vi "Main.vi"() -> ()   [LabVIEW 2018, in "Impedance Tube.lvlib"]
uses:
  Impedance Tube.lvlib
  <vilib>/Analysis/6fits.llb/Remove Outliers (Index).vi
  <vilib>/Analysis/3filter.llb/Savitzky-Golay Filter (DBL).vi
  <vilib>/Utility/config.llb/Read Key (Boolean).vi
  <vilib>/Utility/config.llb/Read Key (Double).vi
  <vilib>/Utility/config.llb/Write Key (Boolean).vi
  <vilib>/Utility/config.llb/Write Key (Double).vi
  <vilib>/Utility/file.llb/Write Delimited Spreadsheet (DBL).vi
  <vilib>/Utility/config.llb/NI_LVConfig.lvlib
  <vilib>/Analysis/NI_AALPro.lvlib
  <vilib>/Analysis/NI_AALBase.lvlib
panel:
  out "Probe Calib Array":cdb[](array[numeric])
  out "max value 2":dbl
  out "max value":i32
  out "error":i32
  out "Filtered Alpha":dbl[](array[numeric])
  out "Normal Specific Impedence Ratio":cdb[](array[numeric])
  out "X Out":dbl[](array[numeric])
  out "Alpha Out":dbl[](array[numeric])
  in  "Mic Calibration":bool
  out "H":cdb[](array[numeric])
  in  "H1":cdb[](array[numeric])
  in  "H2":cdb[](array[numeric])
  in  "Store Params":bool
  in  "Tab Control":T1(tab)
  in  "Mic Device":dbl=4.0
  in  "Speaker Device":dbl
  out "Probe sensitivity ratio":dbl
  out "Upper Freq":dbl
  out "Probe Spacing":dbl
  out "Tube Diameter":dbl
  out "Frequency Spacing":dbl
  out "Speaker Hardware Error":bool
  out "Mic Hardware Error":bool
  out "Calibration Chart  2":dbl[](graph)
  out "Theta":dbl[](graph)
  out "Calibration Chart":cluster{i32, "df":dbl, dbl[]}(graph)
  out "H1 H2":cluster{i32, "df":dbl, "H2":dbl[]}[](graph)
  out "R 2":dbl[](graph)
  out "Alpha 2":cluster{"X Out":dbl[], "Y Out":dbl[]}(graph)
  out "Alpha 3":cluster{"X Out":dbl[], "Y Out":dbl[]}(graph)
  out "H1 H2 3":cluster{i32, dbl, dbl[]}(graph)
  out "R 3":dbl[](graph)
  out "H1 H2 2":cluster{i32, "df":dbl, "H2":dbl[]}[](graph)
  in  "Test Name":string
  in  "OK Button":bool
  out "Outlier Indexes":i32[](array[numeric])
  out "R":cdb[](array[numeric])
  out "Hbar":cdb[](array[numeric])
  in  "Measure":bool
  in  "H(c) 2":cdb[][](array[numeric])
  in  "H(c)":cdb[][](array[numeric])
  in  "output array":dbl[](array[numeric])
  out "Stsarted":bool
  in  "Mic 1 Device":dbl
  out "Mic A Device":dbl
  out "Speaker Volume":dbl
  out "s2 (mm)":dbl
  out "l (mm)":dbl
  out "s (mm)":dbl
  in  "Hardware Sync":bool
  in  "Sample Depth (mm)":dbl
  in  "Density of Air (kg/m3)":dbl
  in  "Speed of Sound m/s":dbl
  in  "Position":bool
  # "Control Panel"
  # "Mic A position"
  # "Position 1 \n(Low Frequency)"
  # "Position 2\n (High Frequency)"
  # "Note: \nSeal the empty mic hole"
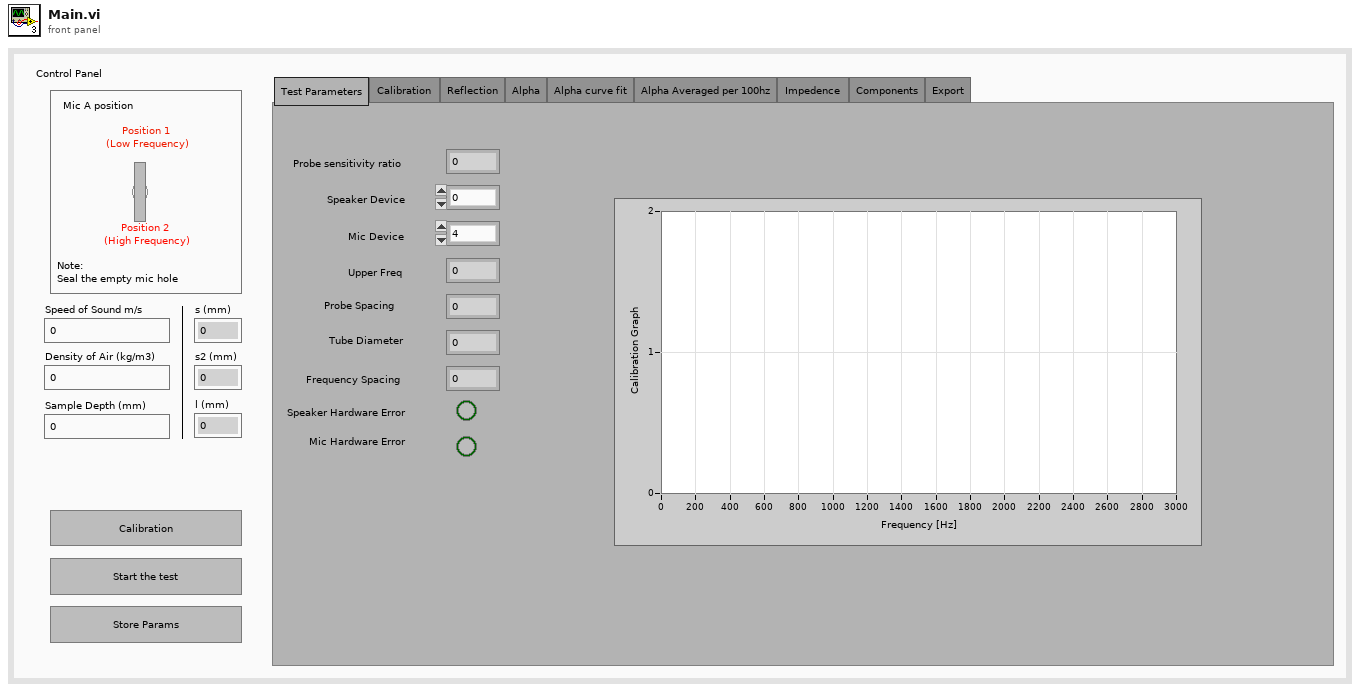
[diagram p1: front panel]
types:
  T1 = enum32{"Test Parameters", "Calibration ", "Reflection", "Alpha", "Alpha curve fit", "Alpha Averaged per 100hz", "Impedence ", "Components", "Export"}
  T2 = enum8{"Enabled", "Disabled", "Disabled and Grayed Out"}
  T3 = enum16{"open", "replace", "create", "open or create", "replace or create", "replace or create with confirmation"}
  T4 = typedef "NI_LVConfig.lvlib/Config Data RefNum.ctl" = refnum<k1>
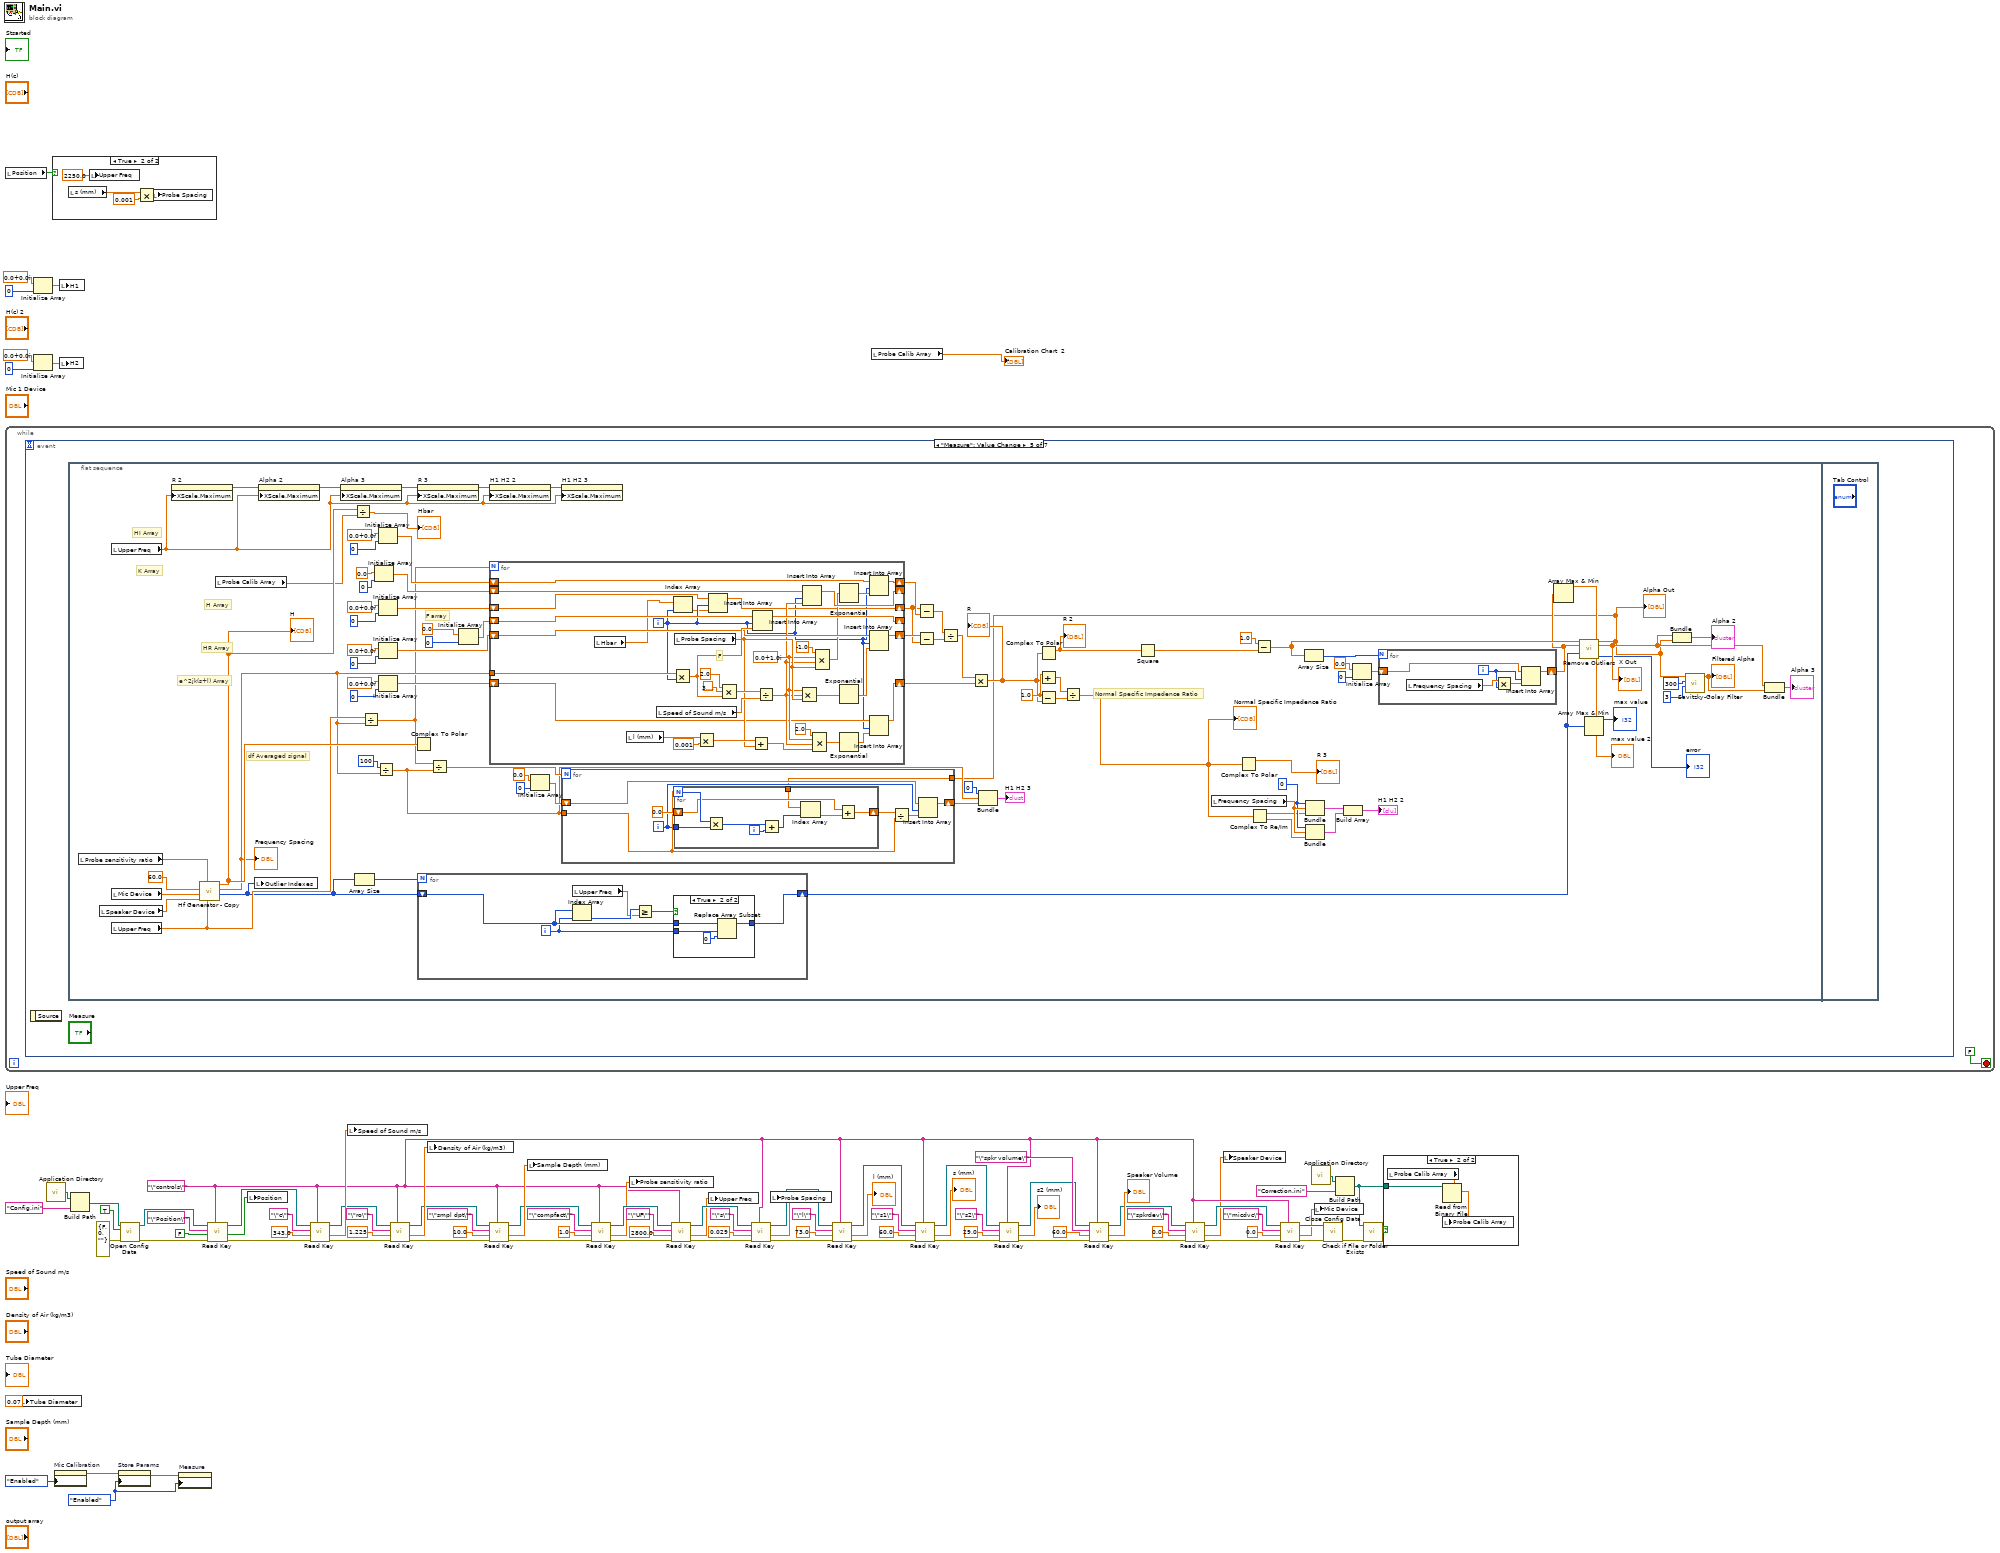
[diagram p0: block diagram]
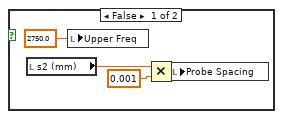
[diagram p2: hidden frame]
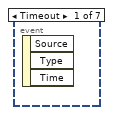
[diagram p4: hidden frame]
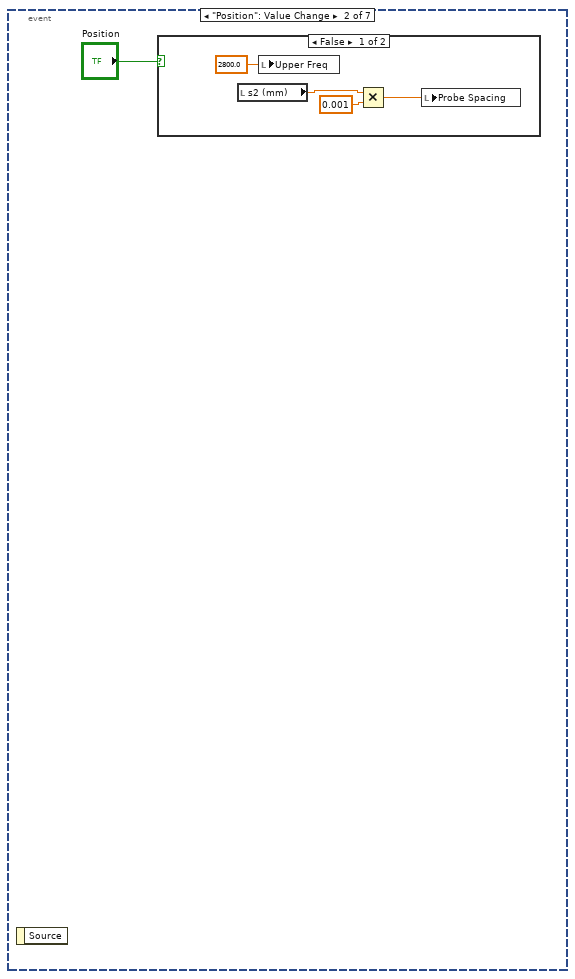
[diagram p5: hidden frame]
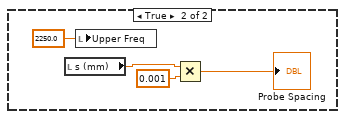
[diagram p6: hidden frame]
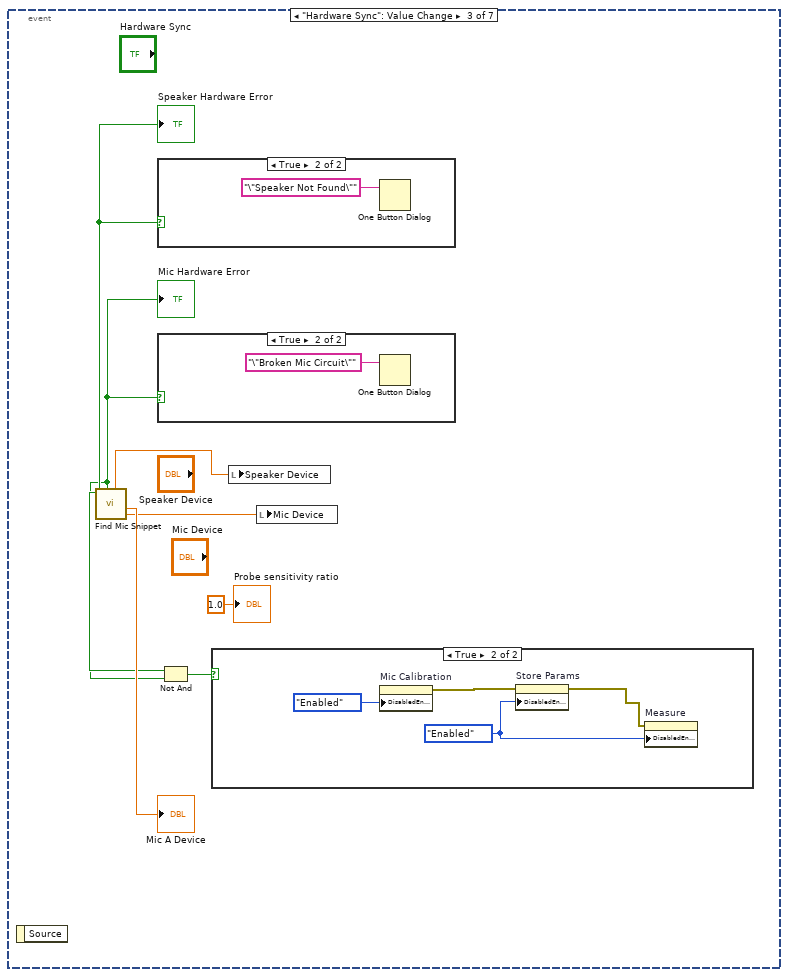
[diagram p7: hidden frame]
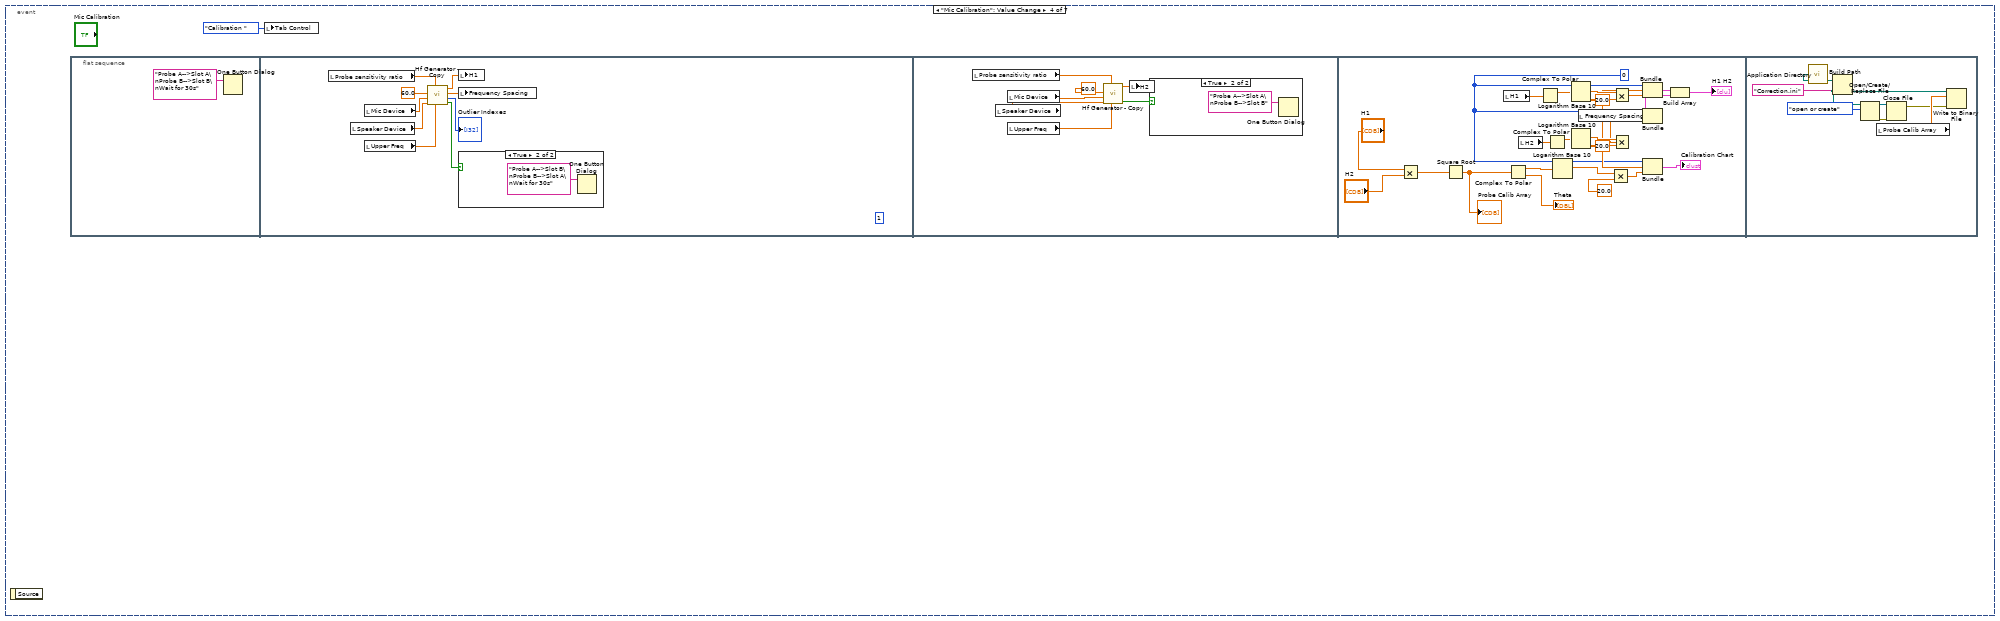
[diagram p11: hidden frame]
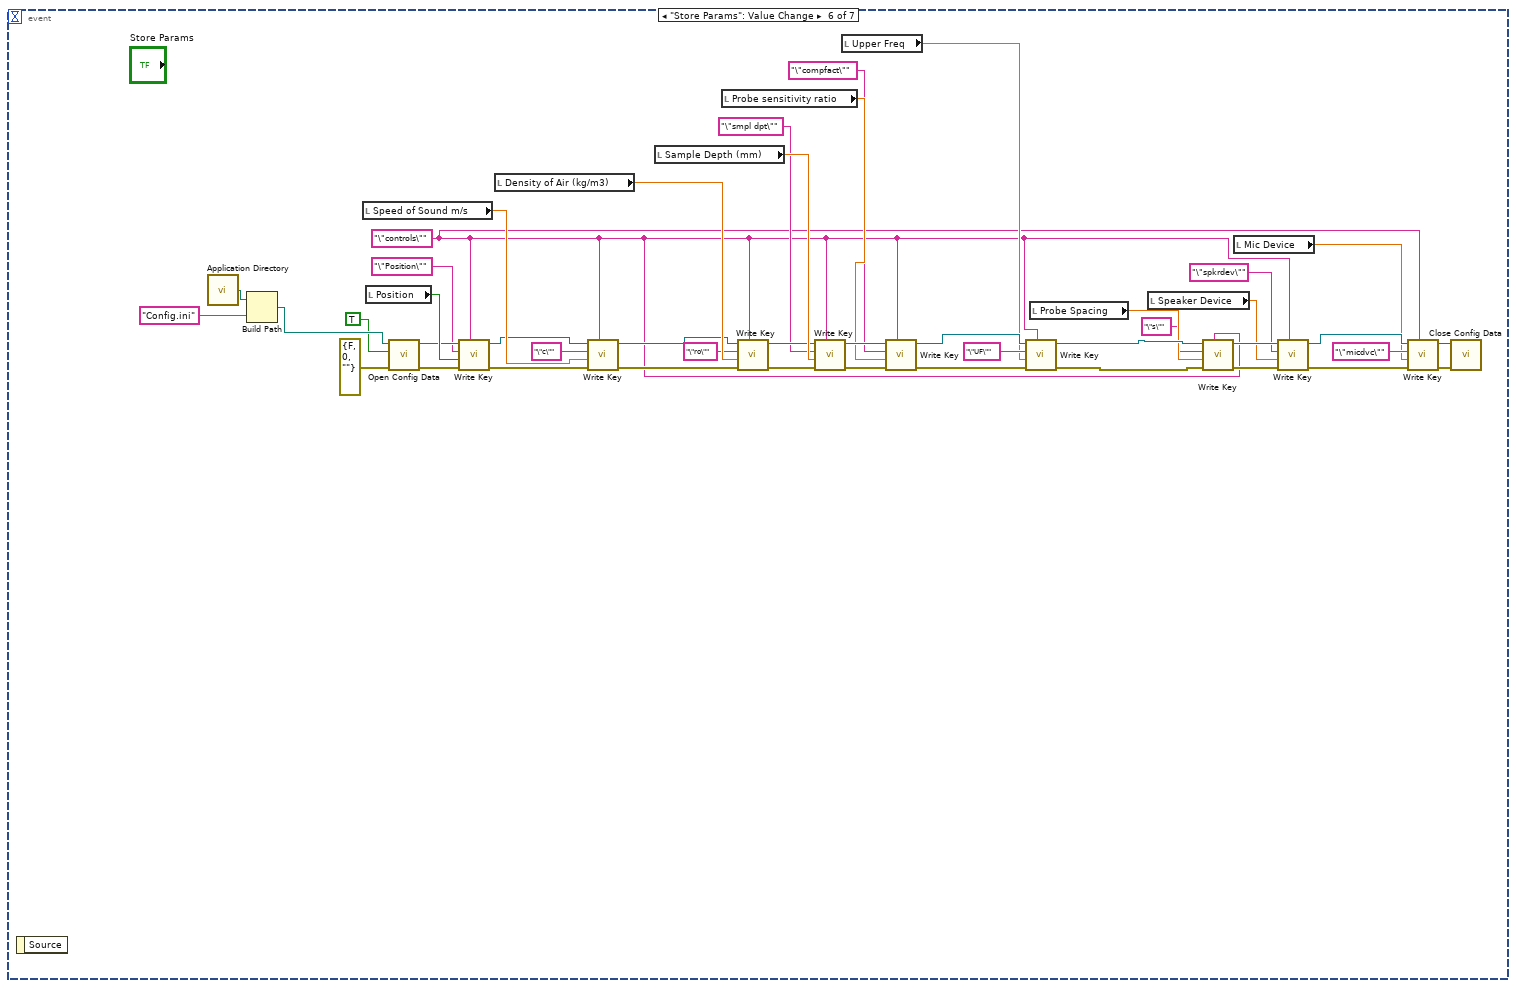
[diagram p15: hidden frame]
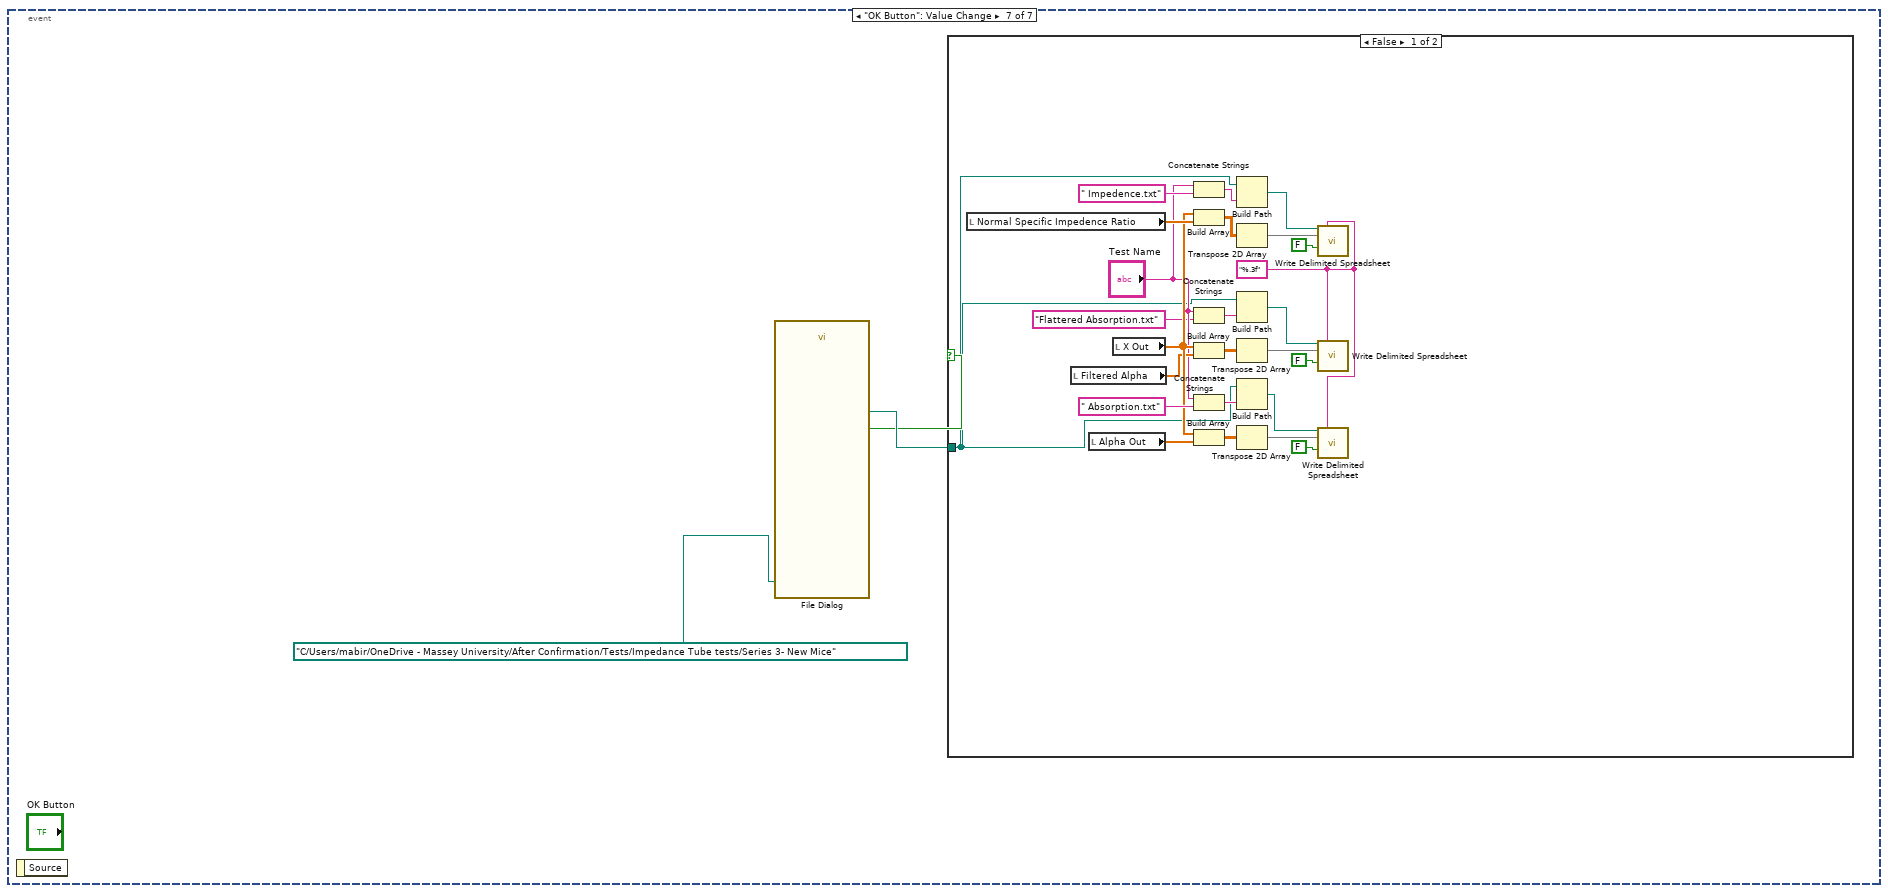
[diagram p16: hidden frame]
diagram:
  w1 = T2."Enabled" ("Disabled")
  w6 = "\"controls\"" ("section")
  n1 = local read "Position"() -> (w34:bool)
  n2 = while {
    stop <- FALSE stop-if-true
    n3 = event shown="[4] \"Measure\": Value Change" {
      selector: _ -> [_ _ _ _ _ _ _]
      dyn-events: _ -> [_ _ _ _ _ _ _]
      timeout: _ -> [_ _ _ _ _ _ _]
      event Timeout {
        n4 = event-data() -> ()  [unwired: 1 in, 3 out]
      }
      event "Position": Value Change {
        n5 = event-data() -> ()  [unwired: 1 in, 1 out]
        n6 = case shown="False" "Position" {
          frame False {
            n7 = local read "s2 (mm)"() -> (w96:dbl)
            n8 = local write "Upper Freq"(2800.0 ("Upper Freq")) -> ()
            n9 = Multiply(x=w96, y=0.001) -> (x*y=w95:dbl)
            n10 = local write "Probe Spacing"(w95) -> ()
          }
          frame True {
            n11 = local read "s (mm)"() -> (w100:dbl)
            n12 = local write "Upper Freq"(2250.0 ("Upper Freq")) -> ()
            n13 = Multiply(x=w100, y=0.001) -> (x*y=→"Probe Spacing":dbl)
          }
        }
      }
      event "Hardware Sync": Value Change {
        n14 = event-data() -> ()  [unwired: 1 in, 1 out]
        n15 = call "Find Mic Snippet.vi"() -> ("Mic B Device"=w103:dbl, "Mic A Device"=→"Mic A Device":dbl, "Speaker Device"=w102:dbl, "Faulty Mic"=w106:bool, "Speaker Not Found"=w107:bool)  [unwired: 3 in, 3 out]
        "Mic Hardware Error" <- w106
        "Speaker Hardware Error" <- w107
        n16 = case shown="True" w107 {
          frame False {
          }
          frame True {
            n17 = One Button Dialog(message="\"Speaker Not Found\"") -> ()  [unwired: 1 in, 1 out]
          }
        }
        n18 = case shown="True" w106 {
          frame False {
          }
          frame True {
            n19 = One Button Dialog(message="\"Broken Mic Circuit\"") -> ()  [unwired: 1 in, 1 out]
          }
        }
        n20 = Not And(1:w106, 2:w107) -> (0:w105:bool)
        n21 = case shown="True" w105 {
          frame False {
          }
          frame True {
            w109 = T2."Enabled" ("Disabled")
            n22 = property on="Mic Calibration" class="Bool"("DisabledEnum"=T2."Enabled" ("Disabled")) -> (error out=w111:errorcluster)  [unwired: 2 in, 1 out]
            n23 = property on="Store Params" class="Bool"(error in=w111, "DisabledEnum"=w109) -> (error out=w110:errorcluster)  [unwired: 1 in, 1 out]
            n24 = property on="Measure" class="Bool"(error in=w110, "DisabledEnum"=w109) -> ()  [unwired: 1 in, 2 out]
          }
        }
        n25 = local write "Speaker Device"(w102) -> ()
        n26 = local write "Mic Device"(w103) -> ()
        "Probe sensitivity ratio" <- 1.0 ("Probe sensitivity ratio")
      }
      event "Mic Calibration": Value Change {
        n27 = event-data() -> ()  [unwired: 1 in, 1 out]
        n28 = flat-sequence {
          frame #0 {
            n29 = One Button Dialog(message="Probe A-->Slot A\nProbe B-->Slot B\nWait for 30s") -> ()  [unwired: 1 in, 1 out]
          }
          frame #1 {
            (unwired) 1 ("Averages")
            n30 = local read "Probe sensitivity ratio"() -> (w122:dbl)
            n31 = local read "Speaker Device"() -> (w124:dbl)
            n32 = local read "Mic Device"() -> (w119:dbl)
            n33 = local read "Upper Freq"() -> (w121:dbl)
            n34 = call "Hf Generator - Copy.vi"("Upper Frequency"=w121, "Mic B Comp Fact"=w122, "Speaker Device"=w124, "Mic B"=w119, "Duration"=60.0) -> ("Done"=w120:bool, "Outlier Indexes"=→"Outlier Indexes":i32[], "df"=w117:dbl, "H(f)"=w123:cdb[])  [unwired: 1 in]
            n35 = local write "H1"(w123) -> ()
            n36 = local write "Frequency Spacing"(w117) -> ()
            n37 = case shown="True" w120 {
              frame False {
              }
              frame True {
                n38 = One Button Dialog(message="Probe A-->Slot B\nProbe B-->Slot A\nWait for 30s") -> ()  [unwired: 1 in, 1 out]
              }
            }
          }
          frame #2 {
            n39 = local read "Probe sensitivity ratio"() -> (w129:dbl)
            n40 = local read "Speaker Device"() -> (w131:dbl)
            n41 = local read "Mic Device"() -> (w133:dbl)
            n42 = local read "Upper Freq"() -> (w127:dbl)
            n43 = call "Hf Generator - Copy.vi"("Upper Frequency"=w127, "Mic B Comp Fact"=w129, "Speaker Device"=w131, "Mic B"=w133, "Duration"=60.0) -> ("Done"=w130:bool, "H(f)"=w128:cdb[])  [unwired: 1 in, 2 out]
            n44 = local write "H2"(w128) -> ()
            n45 = case shown="True" w130 {
              frame False {
              }
              frame True {
                n46 = One Button Dialog(message="Probe A-->Slot A\nProbe B-->Slot B") -> ()  [unwired: 1 in, 1 out]
              }
            }
          }
          frame #3 {
            w148 = 0
            n47 = Multiply(x="H1", y="H2") -> (x*y=w157:cdb[])
            n48 = Square Root(x=w157) -> (sqrt(x)=w135:cdb[])
            "Probe Calib Array" <- w135
            n49 = local read "H1"() -> (w153:cdb[])
            n50 = Complex To Polar(r * e^(i*theta)=w135) -> (r=w145:dbl[], theta=→"Theta":dbl[])
            n51 = local read "H2"() -> (w150:cdb[])
            n52 = Complex To Polar(r * e^(i*theta)=w153) -> (r=w140:dbl[])  [unwired: 1 out]
            n53 = Complex To Polar(r * e^(i*theta)=w150) -> (r=w139:dbl[])  [unwired: 1 out]
            n54 = Logarithm Base 10(1:w145) -> (0:w144:dbl[])
            n55 = Logarithm Base 10(1:w140) -> (0:w155:dbl[])
            n56 = Logarithm Base 10(1:w139) -> (0:w152:dbl[])
            n57 = local read "Frequency Spacing"() -> (w149:dbl)
            n58 = Multiply(x=w144, y=20.0) -> (x*y=w138:dbl[])
            n59 = Multiply(x=w155, y=20.0) -> (x*y=w154:dbl[])
            n60 = Multiply(x=w152, y=20.0) -> (x*y=w151:dbl[])
            n61 = Bundle(w148, "Frequency Spacing"=w149, w154) -> (w147:cluster{i32, "Frequency Spacing":dbl, dbl[]})  [unwired: 1 in]
            n62 = Bundle(w148, "Frequency Spacing"=w149, w151) -> (w146:cluster{i32, "Frequency Spacing":dbl, dbl[]})  [unwired: 1 in]
            n63 = Bundle(w148, "Frequency Spacing"=w149, w138) -> (→"Calibration Chart":cluster{i32, "Frequency Spacing":dbl, dbl[]})  [unwired: 1 in]
            n64 = Build Array(w147, w146) -> (→"H1 H2":cluster{i32, "Frequency Spacing":dbl, dbl[]}[])
          }
          frame #4 {
            n65 = call <vilib>:"Application Directory.vi"() -> ("Application Directory"=w167:path)
            n66 = Build Path(base path=w167, name or relative path="Correction.ini") -> (appended path=w163:path)
            n67 = Open/Create/Replace File(file path (use dialog)=w163, operation (0:open)=T3."open or create") -> (refnum out=w164:refnum<file>, error out=w162:errorcluster)  [unwired: 4 in, 1 out]
            n68 = local read "Probe Calib Array"() -> (w165:cdb[])
            n69 = Close File(refnum=w164, error in=w162) -> (error out=w161:errorcluster)  [unwired: 1 out]
            n70 = Write to Binary File(file (use dialog)=w163, data=w165, error in=w161) -> ()  [unwired: 3 in, 3 out]
          }
        }
        n71 = local write "Tab Control"(T1."Calibration " ("Tab Control")) -> ()
      }
      event "Measure": Value Change {
        n72 = event-data() -> ()  [unwired: 1 in, 1 out]
        n73 = flat-sequence {
          frame #0 {
            w186 = 0
            w192 = 1.0 ("x")
            # "Normal Specific Impedence Ratio"
            # "df Averaged signal"
            # "H Array"
            # "e^2jk(s+l) Array"
            # "HR Array"
            # "HI Array"
            # "K Array"
            # "F array"
            n74 = local read "Probe sensitivity ratio"() -> (w249:dbl)
            n75 = local read "Speaker Device"() -> (w250:dbl)
            n76 = local read "Upper Freq"() -> (w175:dbl)
            n77 = local read "Mic Device"() -> (w251:dbl)
            n78 = local read "Upper Freq"() -> (w244:dbl)
            n79 = property on="R 2" class="WFGraph (strict)"("XScale.Maximum"=w175) -> (error out=w180:errorcluster)  [unwired: 2 in, 1 out]
            n80 = call "Hf Generator - Copy.vi"("Upper Frequency"=w244, "Mic B Comp Fact"=w249, "Speaker Device"=w250, "Mic B"=w251, "Duration"=60.0) -> ("Outlier Indexes"=w199:i32[], "df"=w216:dbl, "H(f)"=w248:cdb[])  [unwired: 1 in, 1 out]
            "H" <- w248
            "Frequency Spacing" <- w216
            n81 = local read "Probe Calib Array"() -> (w247:cdb[])
            n82 = local write "Outlier Indexes"(w199) -> ()
            n83 = property on="Alpha 2" class="XYGraph (strict)"(error in=w180, "XScale.Maximum"=w175) -> (error out=w179:errorcluster)  [unwired: 1 in, 1 out]
            n84 = property on="Alpha 3" class="XYGraph (strict)"(error in=w179, "XScale.Maximum"=w175) -> (error out=w178:errorcluster)  [unwired: 1 in, 1 out]
            n85 = Divide(x=w248, y=w247) -> (x/y=→"Hbar":cdb[])
            n86 = Array Size(array=w199) -> (size(s)=w200:i32)
            n87 = Divide(x=w244, y=w216) -> (x/y=w215:dbl)
            n88 = Initialize Array(0.0 ("element"), 0 ("dimension size")) -> (w240:dbl[])
            n89 = Divide(x=100, y=w216) -> (x/y=w212:dbl)
            n90 = Initialize Array(cdb 0.0+0.0i ("complex element"), 0 ("dimension size")) -> (w235:cdb[])
            n91 = Initialize Array(cdb 0.0+0.0i ("complex element 4"), 0 ("dimension size")) -> (w222:cdb[])
            n92 = Initialize Array(cdb 0.0+0.0i ("complex element 2"), 0 ("dimension size")) -> (w234:cdb[])
            n93 = Initialize Array(cdb 0.0+0.0i ("complex element 3"), 0 ("dimension size")) -> (w231:cdb[])
            n94 = Complex To Polar(r * e^(i*theta)=w248) -> ()  [unwired: 2 out]
            n95 = property on="R 3" class="WFGraph (strict)"(error in=w178, "XScale.Maximum"=w175) -> (error out=w177:errorcluster)  [unwired: 1 in, 1 out]
            n96 = for {
              N: w200 -> [_]
              shift-right: [w253] -> w173
              shift-left: w199 -> [w255]
              i -> [w254]
              n97 = Index Array(array=w255, index=w254) -> (element=w258:i32)
              n98 = local read "Upper Freq"() -> (w257:dbl)
              n99 = Greater Or Equal?(x=w258, y=w257) -> (x >= y?=w256:bool)
              n100 = case shown="True" w256 {
                tunnel: w255 -> [w259 w263]
                tunnel: w254 -> [_ w262]
                tunnel: [w259 w260] -> w253
                frame False {
                }
                frame True {
                  n101 = Replace Array Subset(array=w263, new element=0 ("new element/subarray"), index=w262) -> (w260:i32[])
                }
              }
            }
            n102 = Divide(x=w215, y=w212) -> (x/y=w214:dbl)
            n103 = Initialize Array(0.0 ("element"), 0 ("dimension size")) -> (w243:dbl[])
            n104 = property on="H1 H2 2" class="WFGraph (strict)"(error in=w177, "XScale.Maximum"=w175) -> (error out=w176:errorcluster)  [unwired: 1 in, 1 out]
            n105 = for {
              N: w215 -> [_]
              shift-right: [w320] -> _
              shift-left: w243 -> [w321]
              tunnel: w216 -> [w319]
              shift-right: [w312] -> _
              shift-left: w240 -> [w313]
              shift-right: [w310] -> w230
              shift-left: w235 -> [w311]
              shift-right: [w308] -> w229
              shift-left: w234 -> [w309]
              shift-right: [w291] -> w225
              shift-left: w231 -> [w292]
              shift-right: [w289] -> w221
              shift-left: w222 -> [w290]
              i -> [w288]
              w297 = cdb 0.0+1.0i ("i")
              # "F"
              n106 = local read "Hbar"() -> (w286:cdb[])
              n107 = local read "l (mm)"() -> (w302:dbl)
              n108 = local read "Speed of Sound m/s"() -> (w314:dbl)
              n109 = Multiply(x=w319, y=w288) -> (x*y=w316:dbl)
              n110 = Index Array(array=w286, index=w288) -> (element=w287:cdb)
              n111 = local read "Probe Spacing"() -> (w299:dbl)
              n112 = Multiply(x=w302, y=0.001) -> (x*y=w300:dbl)
              n113 = Insert Into Array(array=w290, index=w288, new element=w287) -> (w289:cdb[])
              n114 = Compound Arithmetic op=MULTIPLY(2.0 ("value"), 3.141592653589793, w316) -> (w315:dbl)
              n115 = Add(x=w300, y=w299) -> (x+y=w295:dbl)
              n116 = Insert Into Array(array=w321, index=w288, new element=w316) -> (w320:dbl[])
              n117 = Divide(x=w315, y=w314) -> (x/y=w296:dbl)
              n118 = Insert Into Array(array=w313, index=w288, new element=w296) -> (w312:dbl[])
              n119 = Compound Arithmetic op=MULTIPLY(w297, w296, w299) -> (w304:cdb)
              n120 = Compound Arithmetic op=MULTIPLY(2.0 ("value"), w297, w296, w295) -> (w294:cdb)
              n121 = Compound Arithmetic op=MULTIPLY(-1.0 ("value"), w297, w296, w299) -> (w306:cdb)
              n122 = Exponential(1:w306) -> (0:w305:cdb)
              n123 = Exponential(1:w304) -> (0:w303:cdb)
              n124 = Exponential(1:w294) -> (0:w293:cdb)
              n125 = Insert Into Array(array=w311, index=w288, new element=w305) -> (w310:cdb[])
              n126 = Insert Into Array(array=w309, index=w288, new element=w303) -> (w308:cdb[])
              n127 = Insert Into Array(array=w292, index=w288, new element=w293) -> (w291:cdb[])
            }
            n128 = Initialize Array(0.0 ("element"), 0 ("dimension size")) -> (w218:dbl[])
            n129 = property on="H1 H2 3" class="WFGraph (strict)"(error in=w176, "XScale.Maximum"=w175) -> ()  [unwired: 1 in, 2 out]
            n130 = Subtract(x=w221, y=w230) -> (x-y=w228:cdb[])
            n131 = Subtract(x=w229, y=w221) -> (x-y=w227:cdb[])
            n132 = Divide(x=w228, y=w227) -> (x/y=w226:cdb[])
            n133 = Multiply(x=w226, y=w225) -> (x*y=w191:cdb[])
            "R" <- w191
            n134 = Add(x=w192, y=w191) -> (x+y=w193:cdb[])
            n135 = Subtract(x=w192, y=w191) -> (x-y=w190:cdb[])
            n136 = Complex To Polar(r * e^(i*theta)=w191) -> (r=w208:dbl[])  [unwired: 1 out]
            "R 2" <- w208
            n137 = Divide(x=w193, y=w190) -> (x/y=w189:cdb[])
            "Normal Specific Impedence Ratio" <- w189
            n138 = Square(x=w208) -> (x^2=w207:dbl[])
            n139 = local read "Frequency Spacing"() -> (w187:dbl)
            n140 = Complex To Polar(r * e^(i*theta)=w189) -> (r=→"R 3":dbl[])  [unwired: 1 out]
            n141 = Complex To Re/Im(x + iy=w189) -> (x=w184:dbl[], y=w185:dbl[])
            n142 = Subtract(x=1.0, y=w207) -> (x-y=w202:dbl[])
            n143 = Array Size(array=w202) -> (size(s)=w206:i32)
            n144 = Bundle(w186, "Frequency Spacing"=w187, w184) -> (w182:cluster{i32, "Frequency Spacing":dbl, dbl[]})  [unwired: 1 in]
            n145 = Bundle(w186, "Frequency Spacing"=w187, w185) -> (w183:cluster{i32, "Frequency Spacing":dbl, dbl[]})  [unwired: 1 in]
            n146 = Build Array(w182, w183) -> (→"H1 H2 2":cluster{i32, "Frequency Spacing":dbl, dbl[]}[])
            n147 = Initialize Array(0.0 ("element"), 0 ("dimension size")) -> (w203:dbl[])
            n148 = for {
              N: w206 -> [_]
              shift-right: [w266] -> w171
              shift-left: w203 -> [w267]
              i -> [w265]
              n149 = local read "Frequency Spacing"() -> (w268:dbl)
              n150 = Multiply(x=w268, y=w265) -> (x*y=w264:dbl)
              n151 = Insert Into Array(array=w267, index=w265, new element=w264) -> (w266:dbl[])
            }
            n152 = Array Max & Min(array=w171) -> (max value=→"max value 2":dbl)  [unwired: 3 out]
            n153 = call-poly <vilib>:"Remove Outliers.vi"("Y"=w202, "X"=w171, "Index"=w173) -> ("Y Out"=w168:dbl[], "X Out"=w198:dbl[], "error"=→"error":i32)  [unwired: 9 in, 1 out]
            "Alpha Out" <- w168
            "X Out" <- w198
            n154 = for {
              N: w214 -> [_]
              shift-right: [w272] -> w213
              shift-left: w218 -> [w273]
              tunnel: w212 -> [w274]
              tunnel: w168 -> [w269]
              i -> [w271]
              n155 = for {
                N: w274 -> [w284]
                tunnel: w271 -> [w285]
                shift-right: [w279] -> w275
                shift-left: 0.0 ("element") -> [w280]
                tunnel: w269 -> [w277]
                i -> [w282]
                n156 = Multiply(x=w284, y=w285) -> (x*y=w283:i32)
                n157 = Add(x=w283, y=w282) -> (x+y=w281:i32)
                n158 = Index Array(array=w277, index=w281) -> (element=w278:dbl)
                n159 = Add(x=w280, y=w278) -> (x+y=w279:dbl)
              }
              n160 = Divide(x=w275, y=w274) -> (x/y=w270:dbl)
              n161 = Insert Into Array(array=w273, index=w271, new element=w270) -> (w272:dbl[])
            }
            n162 = Bundle(0, w212, w213) -> (→"H1 H2 3":cluster{i32, dbl, dbl[]})  [unwired: 1 in]
            n163 = Array Max & Min(array=w173) -> (max value=→"max value":i32)  [unwired: 3 out]
            n164 = Bundle("X Out"=w198, "Y Out"=w168) -> (→"Alpha 2":cluster{"X Out":dbl[], "Y Out":dbl[]})  [unwired: 1 in]
            n165 = call-poly <vilib>:"Savitzky-Golay Filter.vi"("polynomial order"=3, "side points"=300, "X"=w168) -> ("Filtered X"=w197:dbl[])  [unwired: 7 in, 1 out]
            "Filtered Alpha" <- w197
            n166 = Bundle("X Out"=w198, "Filtered X"=w197) -> (→"Alpha 3":cluster{"X Out":dbl[], "Filtered X":dbl[]})  [unwired: 1 in]
          }
          frame #1 {
          }
        }
      }
      event "Store Params": Value Change {
        w326 = "\"controls\"" ("section")
        n167 = event-data() -> ()  [unwired: 1 in, 1 out]
        n168 = call <vilib>:"Application Directory.vi"() -> ("Application Directory"=w365:path)
        n169 = Build Path(base path=w365, name or relative path="Config.ini") -> (appended path=w364:path)
        n170 = local read "Speed of Sound m/s"() -> (w360:dbl)
        n171 = local read "Position"() -> (w363:bool)
        n172 = call <vilib>:"Open Config Data.vi"("error in (no error)"=errorcluster {"status"=FALSE, "code"=0, "source"=""}, "create file if necessary (T)"=TRUE, "configuration file path"=w364) -> ("error out"=w361:errorcluster, "refnum"=w362:T4)  [unwired: 6 in, 1 out]
        n173 = call-poly <vilib>:"Write Key.vi"("section"=w326, "error in (no error)"=w361, "value"=w363, "key"="\"Position\"", "refnum"=w362) -> ("error out"=w359:errorcluster, "refnum out"=w358:T4)  [unwired: 4 in, 1 out]
        n174 = local read "Density of Air (kg/m3)"() -> (w357:dbl)
        n175 = call-poly <vilib>:"Write Key.vi"("section"=w326, "error in (no error)"=w359, "value"=w360, "key"="\"c\"", "refnum"=w358) -> ("error out"=w356:errorcluster, "refnum out"=w355:T4)  [unwired: 4 in, 1 out]
        n176 = local read "Sample Depth (mm)"() -> (w354:dbl)
        n177 = local read "Probe sensitivity ratio"() -> (w350:dbl)
        n178 = call-poly <vilib>:"Write Key.vi"("section"=w326, "error in (no error)"=w356, "value"=w357, "key"="\"ro\"", "refnum"=w355) -> ("error out"=w352:errorcluster, "refnum out"=w353:T4)  [unwired: 4 in, 1 out]
        n179 = call-poly <vilib>:"Write Key.vi"("section"=w326, "error in (no error)"=w352, "value"=w354, "key"="\"smpl dpt\"", "refnum"=w353) -> ("error out"=w349:errorcluster, "refnum out"=w351:T4)  [unwired: 4 in, 1 out]
        n180 = local read "Upper Freq"() -> (w337:dbl)
        n181 = call-poly <vilib>:"Write Key.vi"("section"=w326, "error in (no error)"=w349, "value"=w350, "key"="\"compfact\"", "refnum"=w351) -> ("error out"=w336:errorcluster, "refnum out"=w340:T4)  [unwired: 4 in, 1 out]
        n182 = call-poly <vilib>:"Write Key.vi"("section"=w326, "error in (no error)"=w336, "value"=w337, "key"="\"UF\"", "refnum"=w340) -> ("error out"=w335:errorcluster, "refnum out"=w339:T4)  [unwired: 4 in, 1 out]
        n183 = local read "Probe Spacing"() -> (w334:dbl)
        n184 = local read "Speaker Device"() -> (w322:dbl)
        n185 = call-poly <vilib>:"Write Key.vi"("section"=w326, "error in (no error)"=w335, "value"=w334, "key"="\"s\"", "refnum"=w339) -> ("error out"=w329:errorcluster, "refnum out"=w332:T4)  [unwired: 4 in, 1 out]
        n186 = local read "Mic Device"() -> (w323:dbl)
        n187 = call-poly <vilib>:"Write Key.vi"("section"=w326, "error in (no error)"=w329, "value"=w322, "key"="\"spkrdev\"", "refnum"=w332) -> ("error out"=w328:errorcluster, "refnum out"=w331:T4)  [unwired: 4 in, 1 out]
        n188 = call-poly <vilib>:"Write Key.vi"("section"=w326, "error in (no error)"=w328, "value"=w323, "key"="\"micdvc\"", "refnum"=w331) -> ("error out"=w327:errorcluster, "refnum out"=w330:T4)  [unwired: 4 in, 1 out]
        n189 = call <vilib>:"Close Config Data.vi"("error in (no error)"=w327, "refnum"=w330) -> ()  [unwired: 8 in, 2 out]
      }
      event "OK Button": Value Change {
        n190 = event-data() -> ()  [unwired: 1 in, 1 out]
        n191 = call "File Dialog"("start path"=path "C:/Users/mabir/OneDrive - Massey University/After Confirmation/Tests/Impedance Tube tests/Series 3- New Mice") -> ("selected path"=w368:path, "cancelled"=w367:bool)  [unwired: 11 in, 2 out]
        n192 = case shown="False" w367 {
          tunnel: w368 -> [w370 _]
          frame False {
            w379 = "%.3f" ("format (%.3f)")
            n193 = local read "Normal Specific Impedence Ratio"() -> (w386:cdb[])
            n194 = local read "Filtered Alpha"() -> (w376:dbl[])
            n195 = local read "Alpha Out"() -> (w393:dbl[])
            n196 = local read "X Out"() -> (w377:dbl[])
            n197 = Concatenate Strings("Test Name", " Impedence.txt" ("string")) -> (w381:string)
            n198 = Build Array(w377, w386) -> (w385:cdb[][])
            n199 = Concatenate Strings("Test Name", "Flattered Absorption.txt" ("string")) -> (w371:string)
            n200 = Build Array(w377, w376) -> (w375:dbl[][])
            n201 = Concatenate Strings("Test Name", " Absorption.txt" ("name or relative path")) -> (w387:string)
            n202 = Build Array(w377, w393) -> (w392:dbl[][])
            n203 = Build Path(base path=w370, name or relative path=w381) -> (appended path=w380:path)
            n204 = Transpose 2D Array(2D array=w385) -> (transposed array=w383:cdb[][])
            n205 = Build Path(base path=w370, name or relative path=w371) -> (appended path=w369:path)
            n206 = Transpose 2D Array(2D array=w375) -> (transposed array=w374:dbl[][])
            n207 = Build Path(base path=w370, name or relative path=w387) -> (appended path=w389:path)
            n208 = Transpose 2D Array(2D array=w392) -> (transposed array=w391:dbl[][])
            n209 = call-poly <vilib>:"Write Delimited Spreadsheet.vi"("file path (dialog if empty)"=w380, "format (%.3f)"=w379, "2D data"=w383, "append to file? (new file:F)"=FALSE) -> ()  [unwired: 10 in, 2 out]
            n210 = call-poly <vilib>:"Write Delimited Spreadsheet.vi"("file path (dialog if empty)"=w369, "format (%.3f)"=w379, "2D data"=w374, "append to file? (new file:F)"=FALSE) -> ()  [unwired: 10 in, 2 out]
            n211 = call-poly <vilib>:"Write Delimited Spreadsheet.vi"("file path (dialog if empty)"=w389, "format (%.3f)"=w379, "2D data"=w391, "append to file? (new file:F)"=FALSE) -> ()  [unwired: 10 in, 2 out]
          }
          frame True {
          }
        }
      }
    }
  }
  n212 = local write "Tube Diameter"(0.07 ("diameter")) -> ()
  n213 = Initialize Array(cdb 0.0+0.0i ("element"), 0 ("dimension size")) -> (w39:cdb[])
  n214 = Initialize Array(cdb 0.0+0.0i ("element"), 0 ("dimension size")) -> (w38:cdb[])
  n215 = call <vilib>:"Application Directory.vi"() -> ("Application Directory"=w90:path)
  n216 = case shown="True" w34 {
    frame False {
      n217 = local read "s2 (mm)"() -> (w396:dbl)
      n218 = local write "Upper Freq"(2750.0 ("Upper Freq")) -> ()
      n219 = Multiply(x=w396, y=0.001) -> (x*y=w395:dbl)
      n220 = local write "Probe Spacing"(w395) -> ()
    }
    frame True {
      n221 = local read "s (mm)"() -> (w400:dbl)
      n222 = local write "Upper Freq"(2250.0 ("Upper Freq")) -> ()
      n223 = Multiply(x=w400, y=0.001) -> (x*y=w398:dbl)
      n224 = local write "Probe Spacing"(w398) -> ()
    }
  }
  n225 = property on="Mic Calibration" class="Bool"("DisabledEnum"=T2."Enabled" ("Disabled")) -> (error out=w35:errorcluster)  [unwired: 2 in, 1 out]
  n226 = local write "H1"(w39) -> ()
  n227 = local write "H2"(w38) -> ()
  n228 = Build Path(base path=w90, name or relative path="Config.ini") -> (appended path=w91:path)
  n229 = property on="Store Params" class="Bool"(error in=w35, "DisabledEnum"=w1) -> (error out=w2:errorcluster)  [unwired: 1 in, 1 out]
  n230 = call <vilib>:"Open Config Data.vi"("error in (no error)"=errorcluster {"status"=FALSE, "code"=0, "source"=""}, "create file if necessary (T)"=TRUE, "configuration file path"=w91) -> ("error out"=w87:errorcluster, "refnum"=w83:T4)  [unwired: 6 in, 1 out]
  n231 = property on="Measure" class="Bool"(error in=w2, "DisabledEnum"=w1) -> ()  [unwired: 1 in, 2 out]
  n232 = call-poly <vilib>:"Read Key.vi"("section"=w6, "error in (no error)"=w87, "default value"=FALSE, "key"="\"Position\"", "refnum"=w83) -> ("error out"=w80:errorcluster, "value"=w82:bool, "refnum out"=w81:T4)  [unwired: 3 in, 1 out]
  n233 = local write "Position"(w82) -> ()
  n234 = call-poly <vilib>:"Read Key.vi"("section"=w6, "error in (no error)"=w80, "default value"=343.0, "key"="\"c\"", "refnum"=w81) -> ("error out"=w76:errorcluster, "value"=w78:dbl, "refnum out"=w77:T4)  [unwired: 3 in, 1 out]
  n235 = local write "Speed of Sound m/s"(w78) -> ()
  n236 = call-poly <vilib>:"Read Key.vi"("section"=w6, "error in (no error)"=w76, "default value"=1.225, "key"="\"ro\"", "refnum"=w77) -> ("error out"=w73:errorcluster, "value"=w75:dbl, "refnum out"=w72:T4)  [unwired: 3 in, 1 out]
  n237 = local write "Density of Air (kg/m3)"(w75) -> ()
  n238 = call-poly <vilib>:"Read Key.vi"("section"=w6, "error in (no error)"=w73, "default value"=10.0, "key"="\"smpl dpt\"", "refnum"=w72) -> ("error out"=w19:errorcluster, "value"=w70:dbl, "refnum out"=w21:T4)  [unwired: 3 in, 1 out]
  n239 = local write "Sample Depth (mm)"(w70) -> ()
  n240 = call-poly <vilib>:"Read Key.vi"("section"=w6, "error in (no error)"=w19, "default value"=1.0, "key"="\"compfact\"", "refnum"=w21) -> ("error out"=w18:errorcluster, "value"=w17:dbl, "refnum out"=w20:T4)  [unwired: 3 in, 1 out]
  n241 = local write "Probe sensitivity ratio"(w17) -> ()
  n242 = call-poly <vilib>:"Read Key.vi"("section"=w6, "error in (no error)"=w18, "default value"=2800.0, "key"="\"UF\"", "refnum"=w20) -> ("error out"=w27:errorcluster, "value"=w24:dbl, "refnum out"=w33:T4)  [unwired: 3 in, 1 out]
  n243 = local write "Upper Freq"(w24) -> ()
  n244 = call-poly <vilib>:"Read Key.vi"("section"=w6, "error in (no error)"=w27, "default value"=0.029, "key"="\"s\"", "refnum"=w33) -> ("error out"=w26:errorcluster, "value"=w25:dbl, "refnum out"=w32:T4)  [unwired: 3 in, 1 out]
  n245 = local write "Probe Spacing"(w25) -> ()
  n246 = call-poly <vilib>:"Read Key.vi"("section"=w6, "error in (no error)"=w26, "default value"=73.0, "key"="\"l\"", "refnum"=w32) -> ("error out"=w54:errorcluster, "value"=→"l (mm)":dbl, "refnum out"=w55:T4)  [unwired: 3 in, 1 out]
  n247 = local read "Probe Calib Array"() -> (→"Calibration Chart  2":cdb[])
  n248 = call-poly <vilib>:"Read Key.vi"("section"=w6, "error in (no error)"=w54, "default value"=60.0, "key"="\"s1\"", "refnum"=w55) -> ("error out"=w53:errorcluster, "value"=→"s (mm)":dbl, "refnum out"=w56:T4)  [unwired: 3 in, 1 out]
  n249 = call-poly <vilib>:"Read Key.vi"("section"=w6, "error in (no error)"=w53, "default value"=29.0, "key"="\"s2\"", "refnum"=w56) -> ("error out"=w52:errorcluster, "value"=→"s2 (mm)":dbl, "refnum out"=w57:T4)  [unwired: 3 in, 1 out]
  n250 = call-poly <vilib>:"Read Key.vi"("section"=w6, "error in (no error)"=w52, "default value"=60.0, "key"="\"spkr volume\"", "refnum"=w57) -> ("error out"=w15:errorcluster, "value"=→"Speaker Volume":dbl, "refnum out"=w11:T4)  [unwired: 3 in, 1 out]
  n251 = call-poly <vilib>:"Read Key.vi"("section"=w6, "error in (no error)"=w15, "default value"=0.0, "key"="\"spkrdev\"", "refnum"=w11) -> ("error out"=w16:errorcluster, "value"=w5:dbl, "refnum out"=w13:T4)  [unwired: 3 in, 1 out]
  n252 = local write "Speaker Device"(w5) -> ()
  n253 = call-poly <vilib>:"Read Key.vi"("section"=w6, "error in (no error)"=w16, "default value"=0.0, "key"="\"micdvc\"", "refnum"=w13) -> ("error out"=w14:errorcluster, "value"=w4:dbl, "refnum out"=w12:T4)  [unwired: 3 in, 1 out]
  n254 = call <vilib>:"Application Directory.vi"() -> ("Application Directory"=w47:path)
  n255 = local write "Mic Device"(w4) -> ()
  n256 = call <vilib>:"Close Config Data.vi"("error in (no error)"=w14, "refnum"=w12) -> ("error out"=w45:errorcluster)  [unwired: 8 in, 1 out]
  n257 = Build Path(base path=w47, name or relative path="Correction.ini") -> (appended path=w43:path)
  n258 = call <vilib>:"Check if File or Folder Exists.vi"("error in (no error)"=w45, "path"=w43) -> ("file or folder exists?"=w44:bool)  [unwired: 7 in, 2 out]
  n259 = case shown="True" w44 {
    tunnel: w43 -> [_ w404]
    frame False {
    }
    frame True {
      n260 = local read "Probe Calib Array"() -> (w403:cdb[])
      n261 = Read from Binary File(5:w403, 11:w404) -> (2:w402:cdb[])  [unwired: 4 in, 3 out]
      n262 = local write "Probe Calib Array"(w402) -> ()
    }
  }
